vi "GET_Decision_about_TTL.vi"(10 "Settings cluster":T12 {"Calibration parameters"."True frame time, s" format="%.10g"; "Calibration parameters"."Disp. calibration info"."Speed, µl per ms" format="%.3g"; "Calibration parameters"."True FPS" format="%.10g"; "Calibration parameters"."Timing calibration sw/hw" format="%.10g"; "Conditions presets array"."Specifier(s)"."Validity criteria(s)"."Validity value" min=0.0 step=0.1 format="%.2g"; "Conditions presets array"."Specifier(s)"."Value" step=1.0 format="%#.2g"; "Recording and saving"."Data post-processing"."Order" min=3 max=11 step=2; "Recording and saving"."Data post-processing"."Length" min=5 max=301 step=2; "Geometry"."Cage diameter, mm" scale=0.0..340.0}, 11 "Current animal coordinates and stats":T9 {"Measurements and statistics"."Running, perc. of time" format="%05.2f"}) -> (3 "To be activated":bool[](array[boolean]))   [LabVIEW 2018, in "Tracker.lvlib"]
uses:
  Tracker.lvlib
  Controls/CTL_Settings_cluster.ctl
  Controls/CTL_Histogram_parameters.ctl
  Controls/CTL_Filter_selector.ctl
  Controls/CTL_Acquisition_speed_selector.ctl
  Controls/CTL_Segmented_plot_parameters.ctl
  Controls/CTL_IO_params_cluster.ctl
  Controls/CTL_Conditions_Array.ctl
  Controls/CTL_Conditions_Cluster.ctl
  Controls/CTL_Condition_type.ctl
  Controls/CTL_Comparison_type.ctl
  Controls/CTL_Validity_check_criteria.ctl
  Controls/CTL_Response_info.ctl
  Controls/CTL_Condition_response_type.ctl
  Controls/CTL_Reponse_port_info.ctl
  Controls/CTL_Calibration_parameters.ctl
  Controls/CTL_Dispenser_calibration_info.ctl
  Controls/CTL_Full_data_frame.ctl
  Controls/CTL_Animal_Coordinates_and_Speed.ctl
  Controls/CTL_Measurements_and_Statistics.ctl
  <vilib>/ptbypt/NI_PtbyPt.lvlib
panel:
  out "Conditions presets array":T1 {"Specifier(s)"."Validity criteria(s)"."Validity value" min=0.0 step=0.1 format="%.2g"; "Specifier(s)"."Value" step=1.0 format="%#.2g"}
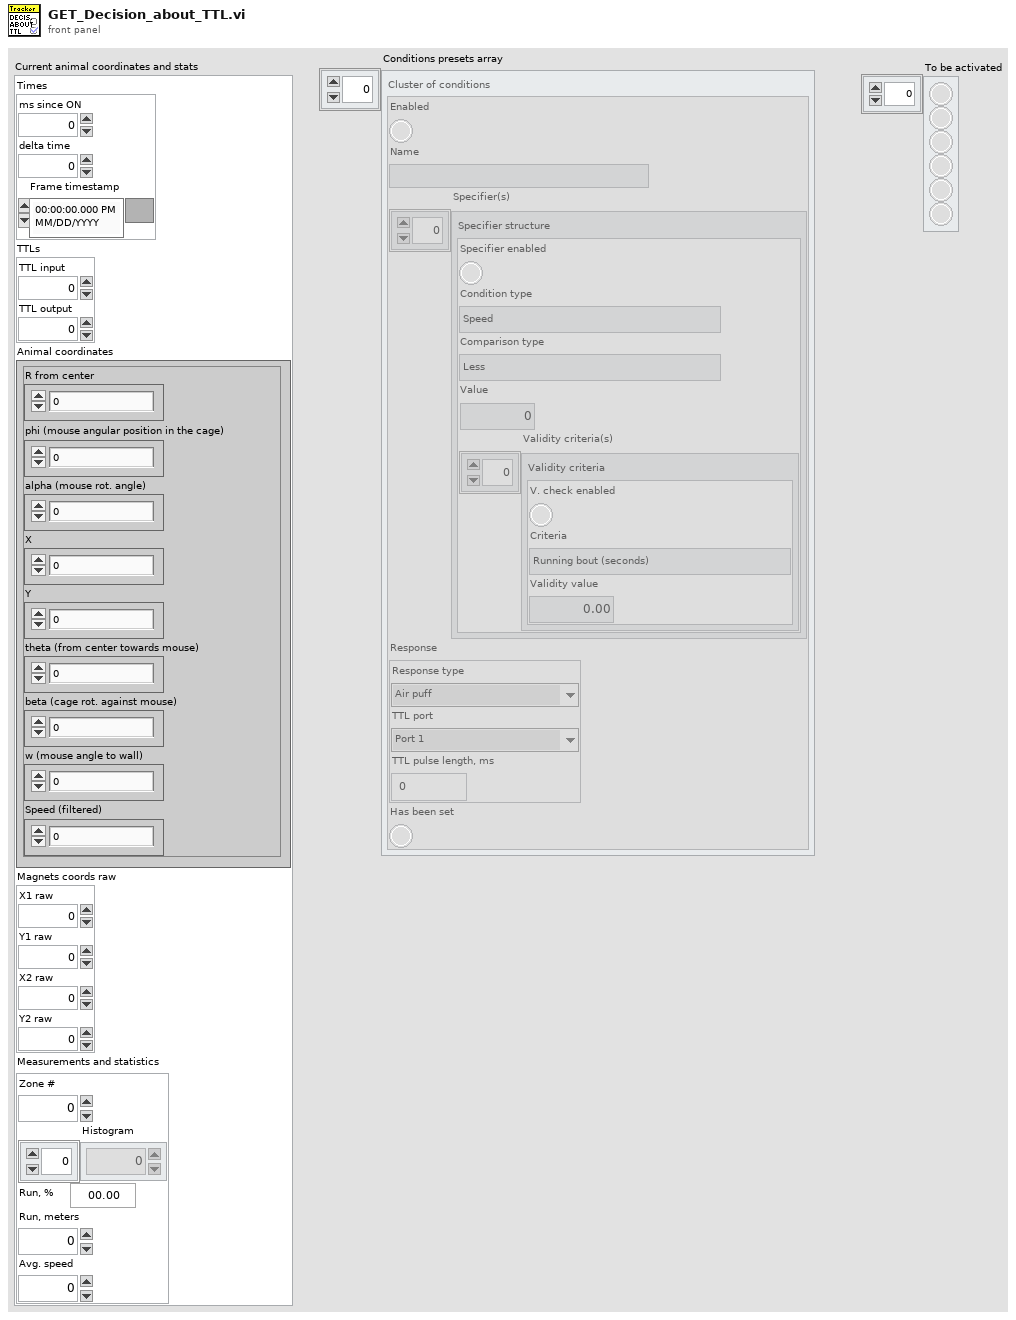
[diagram p1: front panel]
types:
  T1 = typedef "Tracker.lvlib/CTL_Conditions_Array.ctl" = T2[]
  T2 = typedef "Tracker.lvlib/CTL_Conditions_Cluster.ctl" = cluster{"Enabled":bool, "Name":string, "Specifier(s)":cluster{"Specifier enabled":bool, "Condition type":T3, "Comparison type":T4, "Value":dbl, "Validity criteria(s)":cluster{"V. check enabled":bool, "Criteria":T5, "Validity value":dbl}[]}[], "Response":T6, "Has been set":bool}
  T3 = typedef "Tracker.lvlib/CTL_Condition_type.ctl" = enum16{"Speed", "Zone", "Angle to wall"}
  T4 = typedef "Tracker.lvlib/CTL_Comparison_type.ctl" = enum16{"Less", "Less or Equal", "Equal", "Greater or Equal", "Greater", "Not Equal"}
  T5 = typedef "Tracker.lvlib/CTL_Validity_check_criteria.ctl" = enum16{"Running bout (seconds)", "Running bout (meters)"}
  T6 = typedef "Tracker.lvlib/CTL_Response_info.ctl" = cluster{"Response type":T7, "TTL port":T8, "TTL pulse length, ms":dbl}
  T7 = typedef "Tracker.lvlib/CTL_Condition_response_type.ctl" = enum16{"None", "Air puff", "Liquid reward"}
  T8 = typedef "Tracker.lvlib/CTL_Reponse_port_info.ctl" = enum16{"Port 1", "Port 2", "Port 3", "Port 4"}
  T9 = typedef "Tracker.lvlib/CTL_Full_data_frame.ctl" = cluster{"Times":cluster{"ms since ON":u32, "delta time":u32, "Frame timestamp":timestamp}, "TTLs":cluster{"TTL input":i16, "TTL output":i16}, "Animal coordinates":T10, "Magnets coords raw":cluster{"X1 raw":dbl, "Y1 raw":dbl, "X2 raw":dbl, "Y2 raw":dbl}, "Measurements and statistics":T11}
  T10 = typedef "Tracker.lvlib/CTL_Animal_Coordinates_and_Speed.ctl" = cluster{"R from center":dbl, "phi (mouse angular position in the cage)":dbl, "alpha (mouse rot. angle)":dbl, "X":dbl, "Y":dbl, "theta (from center towards mouse)":dbl, "beta (cage rot. against mouse)":dbl, "w (mouse angle to wall)":dbl, "Speed (filtered)":dbl}
  T11 = typedef "Tracker.lvlib/CTL_Measurements_and_Statistics.ctl" = cluster{"Zone #":i8, "Histogram":dbl[], "Running, perc. of time":dbl, "Run, meters":dbl, "Avg. speed":dbl}
  T12 = typedef "Tracker.lvlib/CTL_Settings_cluster.ctl" = cluster{"Defaults":cluster{"Default User":dbl, "VISA Resource Name ":string, "Histogram parameters":T13}, "Recording and saving":cluster{"Researcher name":string, "Name prefix":string, "Data post-processing":T14, "Stop at":dbl, "\"Stop at\" enabled":bool, "Default save folder path":path, "Acquisition FPS":T15}, "Geometry":T16, "IO parameters":T17, "Conditions presets array":T1, "Calibration parameters":T18, "Settings loaded OK":bool}
  T13 = typedef "Tracker.lvlib/CTL_Histogram_parameters.ctl" = cluster{"max":dbl, "min":dbl, "# bins":i32, "threshold":dbl, "thr. type":enum16{"higher accepted", "lower accepted"}}
  T14 = typedef "Tracker.lvlib/CTL_Filter_selector.ctl" = cluster{"Filter type":enum16{"None", "Savitzky-Golay"}, "Length":i32, "Order":i32}
  T15 = typedef "Tracker.lvlib/CTL_Acquisition_speed_selector.ctl" = enum16{"Max", "Optimal", "Eco"}
  T16 = typedef "Tracker.lvlib/CTL_Segmented_plot_parameters.ctl" = cluster{"Cage diameter, mm":u16, "Starting angle MIDFIELD":i16, "Starting angle BORDER":i16, "Radius, mm CENTER":u16, "Radius, mm MIDFIELD":u16, "N segments MIDFIELD":u8, "N segments BORDER":u8, "R-gap, mm":sgl, "Bridge swap":bool, "Bridge H. offset":sgl, "Bridge V. offset":sgl, "Twisted neck":bool, "Alt. magn. orientation":bool, "Sensor board size":enum16{"Small", "Large"}}
  T17 = typedef "Tracker.lvlib/CTL_IO_params_cluster.ctl" = cluster{"IO general config.":u16, "IO 1 configuration":u16, "IO 2 configuration":u16, "IO 3 configuration":u16, "IO 4 configuration":u16, "Activate ext. RS-232":u16, "IO inversion config.":u16, "Sync capability":u8}
  T18 = typedef "Tracker.lvlib/CTL_Calibration_parameters.ctl" = cluster{"Timing calibration sw/hw":dbl, "True FPS":dbl, "True frame time, s":dbl, "Disp. calibration info":T19}
  T19 = typedef "Tracker.lvlib/CTL_Dispenser_calibration_info.ctl" = cluster{"Channel":u8, "Speed, µl per ms":dbl}[]
  T20 = cluster{"Specifier enabled":bool, "Condition type":T3, "Comparison type":T4, "Value":dbl, "Validity criteria(s)":cluster{"V. check enabled":bool, "Criteria":T5, "Validity value":dbl}[]}[]
  T21 = cluster{"V. check enabled":bool, "Criteria":T5, "Validity value":dbl}[]
  T22 = cluster{"V. check enabled":bool, "Criteria":T5, "Validity value":dbl}
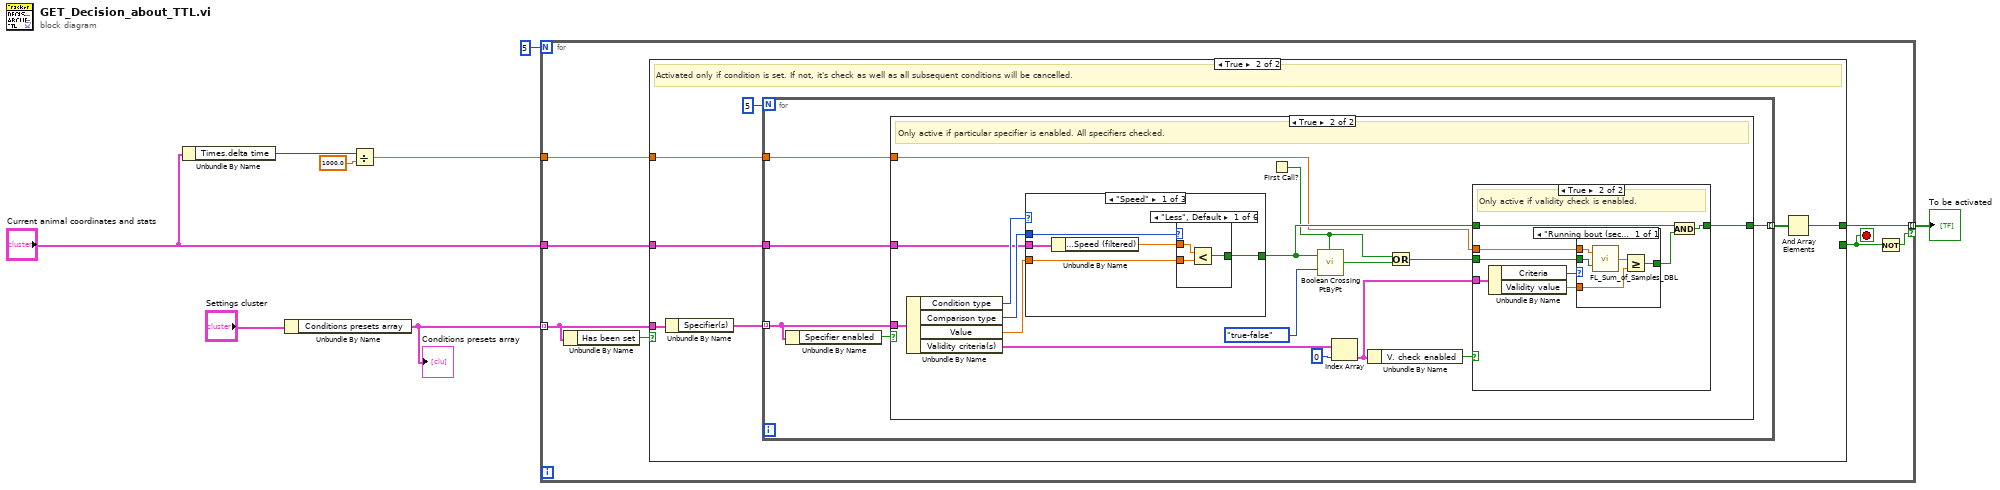
[diagram p0: block diagram]
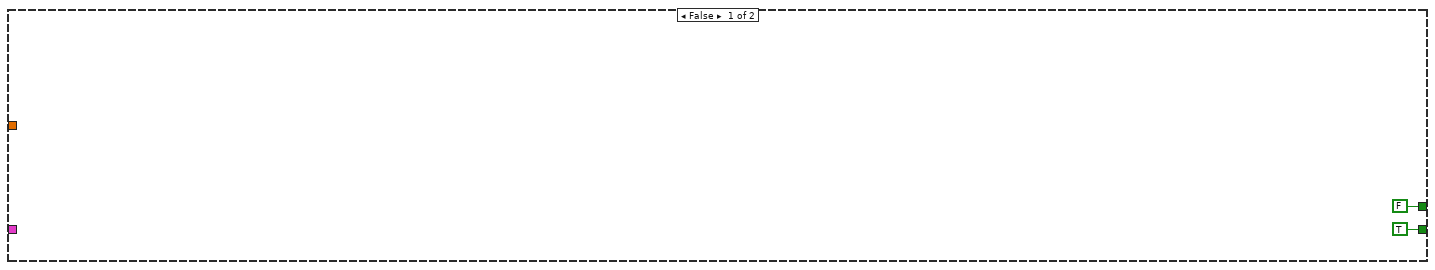
[diagram p2: hidden frame]
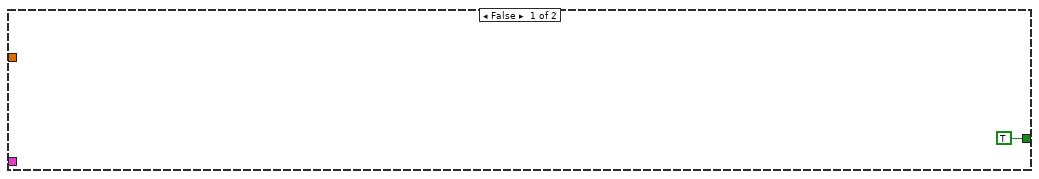
[diagram p3: hidden frame]
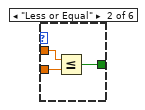
[diagram p4: hidden frame]
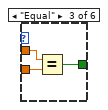
[diagram p5: hidden frame]
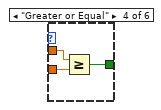
[diagram p6: hidden frame]
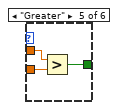
[diagram p7: hidden frame]
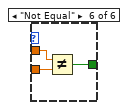
[diagram p8: hidden frame]
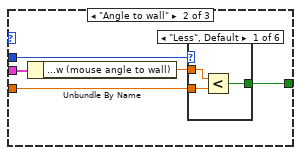
[diagram p9: hidden frame]
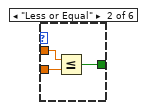
[diagram p10: hidden frame]
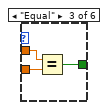
[diagram p11: hidden frame]
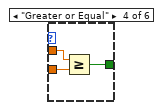
[diagram p12: hidden frame]
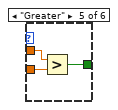
[diagram p13: hidden frame]
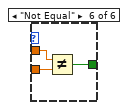
[diagram p14: hidden frame]
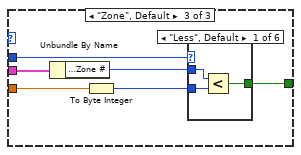
[diagram p15: hidden frame]
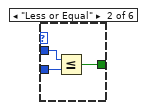
[diagram p16: hidden frame]
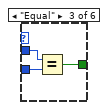
[diagram p17: hidden frame]
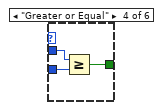
[diagram p18: hidden frame]
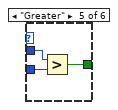
[diagram p19: hidden frame]
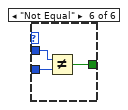
[diagram p20: hidden frame]
diagram:
  n1 = Unbundle By Name("Current animal coordinates and stats") -> ("Times.delta time"=w3:u32)
  n2 = Unbundle By Name("Settings cluster") -> ("Conditions presets array"=w7:T1)
  "Conditions presets array" <- w7
  n3 = Divide(x=w3, y=1000.0) -> (x/y=w1:dbl)
  n4 = for {
    N: 5 -> [_]
    tunnel: w7 -> [w15] mode=indexing
    tunnel: [w13] -> w5 mode=indexing if=w9
    tunnel: "Current animal coordinates and stats" -> [w12]
    tunnel: w1 -> [w11]
    stop <- w10 stop-if-true
    n5 = Unbundle By Name(w15) -> ("Has been set"=w14:bool)
    n6 = case shown="True" w14 {
      tunnel: w15 -> [_ w24]
      tunnel: [TRUE _] -> w10
      tunnel: [FALSE w20] -> w13
      tunnel: w12 -> [_ w19]
      tunnel: w11 -> [_ w18]
      frame False {
      }
      frame True {
        # "Activated only if condition is set. If not, it's check as well as all subsequent conditions will be cancelled."
        n7 = Unbundle By Name(w24) -> ("Specifier(s)"=w22:T20)
        n8 = for {
          N: 5 -> [_]
          tunnel: w22 -> [w28] mode=indexing
          tunnel: [w27] -> w21 mode=indexing
          tunnel: w19 -> [w26]
          tunnel: w18 -> [w25]
          n9 = Unbundle By Name(w28) -> ("Specifier enabled"=w29:bool)
          n10 = case shown="True" w29 {
            tunnel: w28 -> [_ w46]
            tunnel: [TRUE w38] -> w27
            tunnel: w26 -> [_ w37]
            tunnel: w25 -> [_ w31]
            frame False {
            }
            frame True {
              # "Only active if particular specifier is enabled. All specifiers checked."
              n11 = Unbundle By Name(w46) -> ("Condition type"=w43:T3, "Comparison type"=w40:T4, "Value"=w41:dbl, "Validity criteria(s)"=w45:T21)
              n12 = case shown="\"Speed\"" w43 {
                tunnel: w37 -> [w51 w74 w98]
                tunnel: w41 -> [w49 w72 w96]
                tunnel: w40 -> [w48 w71 w95]
                tunnel: [w47 w70 w93] -> w36
                frame "Speed" {
                  n13 = Unbundle By Name(w51) -> ("Animal coordinates.Speed (filtered)"=w50:dbl)
                  n14 = case shown="\"Less\", Default" w48 {
                    tunnel: w50 -> [w54 w57 w60 w63 w66 w69]
                    tunnel: [w53 w56 w59 w62 w65 w68] -> w47
                    tunnel: w49 -> [w52 w55 w58 w61 w64 w67]
                    frame "Less", Default {
                      n15 = Less?(x=w54, y=w52) -> (x < y?=w53:bool)
                    }
                    frame "Less or Equal" {
                      n16 = Less Or Equal?(x=w57, y=w55) -> (x <= y?=w56:bool)
                    }
                    frame "Equal" {
                      n17 = Equal?(x=w60, y=w58) -> (x = y?=w59:bool)
                    }
                    frame "Greater or Equal" {
                      n18 = Greater Or Equal?(x=w63, y=w61) -> (x >= y?=w62:bool)
                    }
                    frame "Greater" {
                      n19 = Greater?(x=w66, y=w64) -> (0:w65:bool)
                    }
                    frame "Not Equal" {
                      n20 = Not Equal?(x=w69, y=w67) -> (x != y?=w68:bool)
                    }
                  }
                }
                frame "Angle to wall" {
                  n21 = Unbundle By Name(w74) -> ("Animal coordinates.w (mouse angle to wall)"=w73:dbl)
                  n22 = case shown="\"Less\", Default" w71 {
                    tunnel: w73 -> [w77 w80 w83 w86 w89 w92]
                    tunnel: [w76 w79 w82 w85 w88 w91] -> w70
                    tunnel: w72 -> [w75 w78 w81 w84 w87 w90]
                    frame "Less", Default {
                      n23 = Less?(x=w77, y=w75) -> (x < y?=w76:bool)
                    }
                    frame "Less or Equal" {
                      n24 = Less Or Equal?(x=w80, y=w78) -> (x <= y?=w79:bool)
                    }
                    frame "Equal" {
                      n25 = Equal?(x=w83, y=w81) -> (x = y?=w82:bool)
                    }
                    frame "Greater or Equal" {
                      n26 = Greater Or Equal?(x=w86, y=w84) -> (x >= y?=w85:bool)
                    }
                    frame "Greater" {
                      n27 = Greater?(x=w89, y=w87) -> (0:w88:bool)
                    }
                    frame "Not Equal" {
                      n28 = Not Equal?(x=w92, y=w90) -> (x != y?=w91:bool)
                    }
                  }
                }
                frame "Zone", Default {
                  n29 = Unbundle By Name(w98) -> ("Measurements and statistics.Zone #"=w97:i8)
                  n30 = To Byte Integer(number=w96) -> (8bit integer=w94:i8)
                  n31 = case shown="\"Less\", Default" w95 {
                    tunnel: w97 -> [w101 w104 w107 w110 w113 w116]
                    tunnel: [w100 w103 w106 w109 w112 w115] -> w93
                    tunnel: w94 -> [w99 w102 w105 w108 w111 w114]
                    frame "Less", Default {
                      n32 = Less?(x=w101, y=w99) -> (x < y?=w100:bool)
                    }
                    frame "Less or Equal" {
                      n33 = Less Or Equal?(x=w104, y=w102) -> (x <= y?=w103:bool)
                    }
                    frame "Equal" {
                      n34 = Equal?(x=w107, y=w105) -> (x = y?=w106:bool)
                    }
                    frame "Greater or Equal" {
                      n35 = Greater Or Equal?(x=w110, y=w108) -> (x >= y?=w109:bool)
                    }
                    frame "Greater" {
                      n36 = Greater?(x=w113, y=w111) -> (0:w112:bool)
                    }
                    frame "Not Equal" {
                      n37 = Not Equal?(x=w116, y=w114) -> (x != y?=w115:bool)
                    }
                  }
                }
              }
              n38 = First Call?() -> (First Call?: T/F=w32:bool)
              n39 = call <vilib>:"Boolean Crossing PtByPt.vi"("initialize"=w32, "direction"=enum16{"either", "false-true", "true-false"}."true-false", "input"=w36) -> ("crossing"=w34:bool)
              n40 = Index Array(array=w45, index=0) -> (element=w39:T22)
              n41 = Unbundle By Name(w39) -> ("V. check enabled"=w42:bool)
              n42 = Or(x=w32, y=w34) -> (x .or. y?=w33:bool)
              n43 = case shown="True" w42 {
                tunnel: w36 -> [w117 w121]
                tunnel: [w117 w122] -> w38
                tunnel: w39 -> [_ w125]
                tunnel: w33 -> [_ w120]
                tunnel: w31 -> [_ w118]
                frame False {
                }
                frame True {
                  # "Only active if validity check is enabled."
                  n44 = Unbundle By Name(w125) -> ("Criteria"=w124:T5, "Validity value"=w123:dbl)
                  n45 = case shown="\"Running bout (seconds)\", Default" w124 {
                    tunnel: w123 -> [w130]
                    tunnel: w120 -> [w126]
                    tunnel: [w129] -> w119
                    tunnel: w118 -> [w128]
                    frame "Running bout (seconds)", Default {
                      n46 = call "FL_Sum_of_Samples_DBL.vi"("Reset?"=w126, "Input sample"=w128) -> ("Sum of samples"=w127:dbl)
                      n47 = Greater Or Equal?(x=w127, y=w130) -> (x >= y?=w129:bool)
                    }
                  }
                  n48 = And(x=w121, y=w119) -> (x .and. y?=w122:bool)
                }
              }
            }
          }
        }
        n49 = And Array Elements(Boolean array=w21) -> (logical AND=w20:bool)
      }
    }
    n50 = Not(x=w10) -> (.not. x?=w9:bool)
  }
  "To be activated" <- w5
